vi "Incoming Bit.vi"(8 "error in (no error)":errorcluster, 10 "Set/Reset":bool, 11 "Controller in":refnum<class "Controller.lvclass">) -> (0 "error out":errorcluster, 3 "Controller out":refnum<class "Controller.lvclass">)   [LabVIEW 2022 SP3, in "Controller.lvlib" / "Controller.lvclass"]
uses:
  Controller.lvclass
  Controller.lvclass/Controller.ctl
  Controller -- Sig Acq Interface Messages/Incoming Bit Msg/Incoming Bit Msg.lvclass
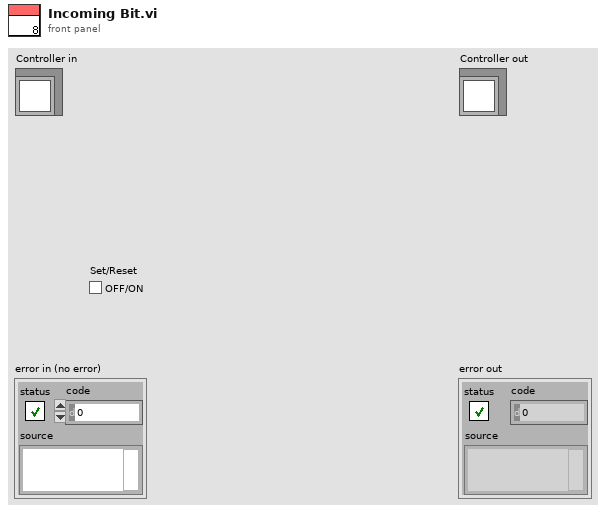
[diagram p1: front panel]
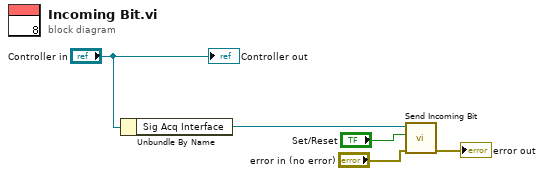
[diagram p0: block diagram]
diagram:
  n1 = Unbundle By Name("Controller in") -> ("Sig Acq Interface"=w4:refnum<class "Message Enqueuer.lvclass">)
  n2 = call "Send Incoming Bit.vi"("error in (no error)"="error in (no error)", "Set/Reset"="Set/Reset", "Message Enqueuer"=w4) -> ("error out"=→"error out":errorcluster)  [unwired: 7 in, 1 out]
  "Controller out" <- "Controller in"
